vi "labview-client.vi"() -> ()   [LabVIEW 2019]
uses:
  <vilib>/addons/zeromq/socket_type.ctl
  <vilib>/addons/zeromq/endpoint_proto.ctl
  <vilib>/addons/zeromq/zmq_context.lvclass
  <vilib>/addons/zeromq/zmq_socket.lvclass
  <vilib>/addons/zeromq/zeromq.lvlib
panel:
  in  "address":string="127.0.0.1"
  in  "port":u16=5555
  out "TCP address":string="tcp://127.0.0.1:5555"
  in  "command":string="test()"
  out "data":string
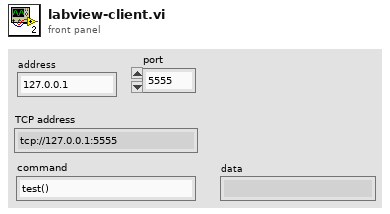
[diagram p1: front panel]
types:
  T1 = typedef "zeromq.lvlib/endpoint_proto.ctl" = enum16{"tcp", "udp", "inproc"}
  T2 = typedef "zeromq.lvlib/socket_type.ctl" = enum8{"ZMQ_PAIR", "ZMQ_PUB", "ZMQ_SUB", "ZMQ_REQ", "ZMQ_REP", "ZMQ_DEALER", "ZMQ_ROUTER", "ZMQ_PULL", "ZMQ_PUSH", "ZMQ_XPUB", "ZMQ_XSUB", "ZMQ_STREAM", "ZMQ_SERVER", "ZMQ_CLIENT", "ZMQ_RADIO", "ZMQ_DISH", "ZMQ_GATHER", "ZMQ_SCATTER", "ZMQ_DGRAM"}
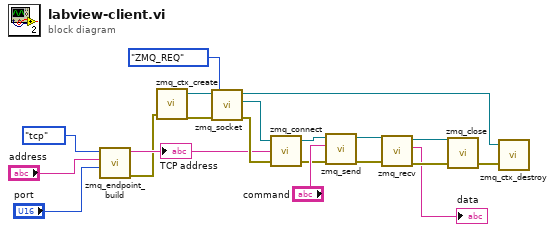
[diagram p0: block diagram]
diagram:
  n1 = call <vilib>:"zmq_endpoint_build.vi"("port"="port", "address"="address", "protocol (tcp)"=endpoint_proto."tcp") -> ("error out"=w1:errorcluster, "endpoint"=w4:string)  [unwired: 2 in, 1 out]
  "TCP address" <- w4
  n2 = call <vilib>:"zmq_ctx_create.vi"("error in"=w1) -> ("error out"=w19:errorcluster, "context out"=w20:refnum<class "zmq_context.lvclass">)  [unwired: 3 in]
  n3 = call <vilib>:"zmq_socket.vi"("error in"=w19, "socket type"=socket_type."ZMQ_REQ", "context in"=w20) -> ("error out"=w16:errorcluster, "socket out"=w17:refnum<class "zmq_socket.lvclass">, "context out"=w8:refnum<class "zmq_context.lvclass">)  [unwired: 2 in]
  n4 = call <vilib>:"zmq_connect.vi"("error in"=w16, "endpoint"=w4, "socket in"=w17) -> ("error out"=w14:errorcluster, "socket out"=w13:refnum<class "zmq_socket.lvclass">)  [unwired: 1 in]
  n5 = call <vilib>:"zmq_send.vi"("error in"=w14, "data"="command", "socket in"=w13) -> ("error out"=w12:errorcluster, "socket out"=w11:refnum<class "zmq_socket.lvclass">)  [unwired: 4 in]
  n6 = call <vilib>:"zmq_recv.vi"("error in"=w12, "socket in"=w11) -> ("error out"=w10:errorcluster, "data"=→"data":string, "socket out"=w6:refnum<class "zmq_socket.lvclass">)  [unwired: 3 in, 2 out]
  n7 = call <vilib>:"zmq_close.vi"("error in"=w10, "socket"=w6) -> ("error out"=w9:errorcluster)  [unwired: 3 in]
  n8 = call <vilib>:"zmq_ctx_destroy.vi"("error in"=w9, "context in"=w8) -> ()  [unwired: 3 in, 1 out]
